vi "SetDualPassMode.vi"(0 "Mode":T2 items=["[read only]"=-2147483648, "Feedback"=0, "First Line Profile"=1], 5 "error in":T1) -> (14 "Mode out":T2 items=["[read only]"=-2147483648, "Feedback"=0, "First Line Profile"=1], 19 "error out":T1)   [LabVIEW 2016]
doc: "Two modes are available for the Dual Pass. The first is feedback (mode = 0) and the second one is first line profile (mode = 1)."
uses:
  Controls/Dual-Pass-Feedback-Mode_Selection.ctl
  Controls/Error_Out.ctl
  Files_ASC500/DLL/ASC500_RemoteControlV27.dll
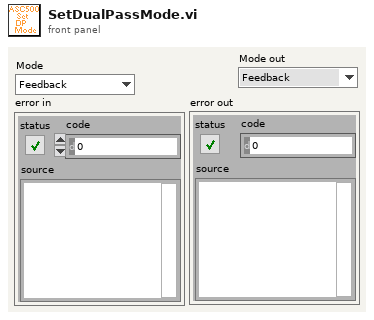
[diagram p1: front panel]
types:
  T1 = typedef "Error_Out.ctl" = errorcluster
  T2 = typedef "Dual-Pass-Feedback-Mode_Selection.ctl" = i32
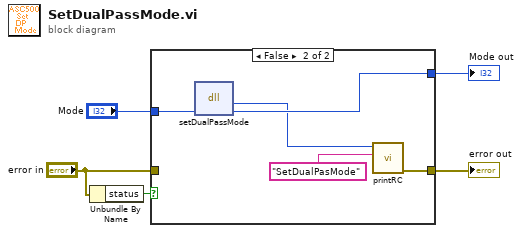
[diagram p0: block diagram]
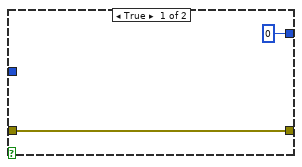
[diagram p2: hidden frame]
diagram:
  n1 = Unbundle By Name("error in") -> ("status"=w5:bool)
  n2 = case shown="False" w5 {
    tunnel: [w6 w10] -> w4
    tunnel: "Mode" -> [_ w12]
    tunnel: [0 ("Mode") w11] -> w2
    tunnel: "error in" -> [w6 _]
    frame True {
    }
    frame False {
      n3 = dll-call lib="G:/SCMOperations/Share/ELE/Produkt Information/ASC500/04 Remote Control/02 development versions/2018Nov06/Files_ASC500/DLL/ASC500_RemoteControlV27.dll" fn="setDualPassMode"("Mode"=w12) -> ("return type"=w9:i32, "Mode"=w11:i32)  [unwired: 3 in, 2 out]
      n4 = call "printRC.vi"("additional information"="SetDualPasMode", "RC"=w9) -> ("error out"=w10:T1)  [unwired: 9 in]
    }
  }
  "error out" <- w4
  "Mode out" <- w2
